vi "Panel.vi"(8 "error in (no error)":errorcluster, 10 "VI Panel Path":path, 11 "Panel in":refnum<class "Panel.lvclass">) -> (0 "error out":errorcluster, 3 "Panel out":refnum<class "Panel.lvclass">)   [LabVIEW 2019, in "Panel.lvclass"]
uses:
  Panel.lvclass
  Panel.lvclass/Panel.ctl
  setVIName.vi
  setReference.vi
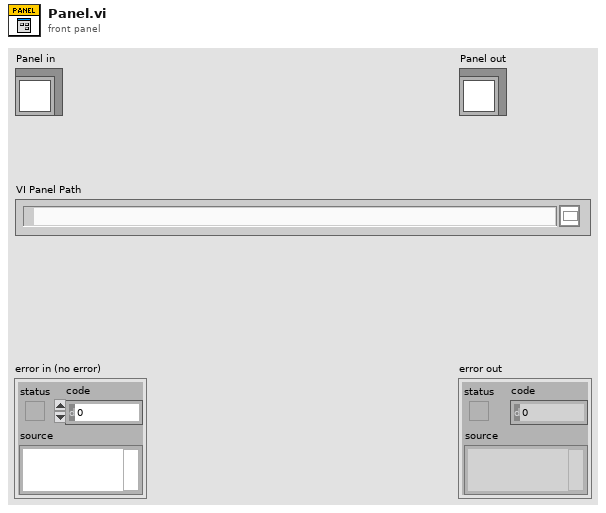
[diagram p1: front panel]
types:
  T1 = enum16{"Open Reference", "Launch VI", "Get VI Outputs"}
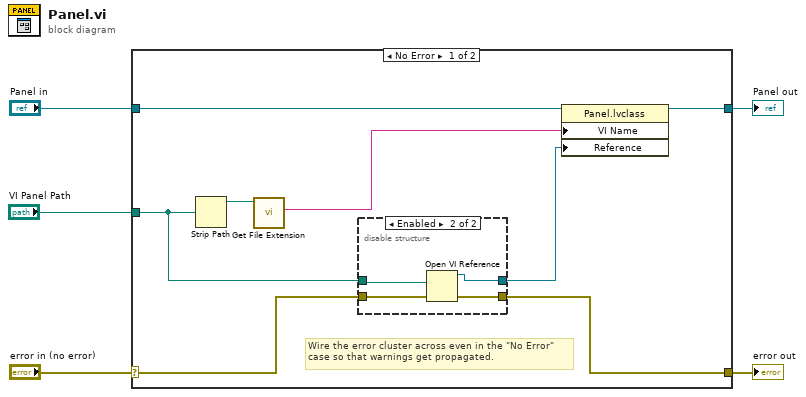
[diagram p0: block diagram]
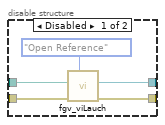
[diagram p2: hidden frame]
diagram:
  n1 = case shown="No Error" "error in (no error)" {
    selector: "error in (no error)" -> [w9 w24]
    tunnel: [w8 w24] -> w4
    tunnel: [w12 w23] -> w2
    tunnel: "Panel in" -> [w13 w23]
    tunnel: "VI Panel Path" -> [w7 _]
    frame No Error {
      # "Wire the error cluster across even in the \"No Error\"\ncase so that warnings get propagated."
      n2 = Strip Path(path=w7) -> (stripped path=w11:path)  [unwired: 1 out]
      n3 = call <vilib>:"Get File Extension.vi"("file"=w11) -> ("lowercase file extension"=w10:string)  [unwired: 6 in, 4 out]
      n4 = disable-structure shown="Enabled" {
        disable-tunnel: w9 -> [w18 w21]
        disable-tunnel: [w17 w19] -> w8
        disable-tunnel: w7 -> [w16 w22]
        disable-tunnel: [w14 w20] -> w6
        frame Disabled {
          n5 = call "fgv_viLauch.vi"("Option"=T1."Open Reference", "Error In"=w18, "vi path"=w16) -> ("Error Out"=w17:errorcluster, "VI ref Out"=w14:refnum<vi>)  [unwired: 6 in, 1 out]
        }
        frame Enabled {
          n6 = Open VI Reference(vi path=w22, error in (no error)=w21) -> (vi reference=w20:refnum<vi>, error out=w19:errorcluster)  [unwired: 4 in]
        }
      }
      n7 = property class="Panel.lvclass"(reference=w13, "VI Name"=w10, "Reference"=w6) -> (reference out=w12:refnum<class "Panel.lvclass">)  [unwired: 1 in, 1 out]
    }
    frame Error {
    }
  }
  "error out" <- w4
  "Panel out" <- w2
